vi "Create Menu Options.vi"(6 "Variant in":variant, 7 "Shift Pressed?":bool, 8 "error in (no error)":errorcluster, 10 "QD Combo Box Ref":refnum<vi>, 11 "QD Launch VI Ref":refnum<vi>) -> (0 "error out":errorcluster, 4 "Variant out":variant)   [LabVIEW 2020]
doc: "PLUGIN_DESCRIPTION: Allows you to perform all the options in the right-click > Create... menu with your keyboard. You can perform these operations with one or more objects selected.\n\nSupported options: local, reference, property, invoke, control, indicator, constant\n\nNote: there are a number of \"shorthand\" commands recognized for each object type. For example, you could type ctl instead of control. View the diagram of the plugin VI to see all supported shorthand commands (or add your own).\n\nPLUGIN_DEFAULT_SHORTCUT: a"
panel:
  in  "Undo Name":string="Object Creation"
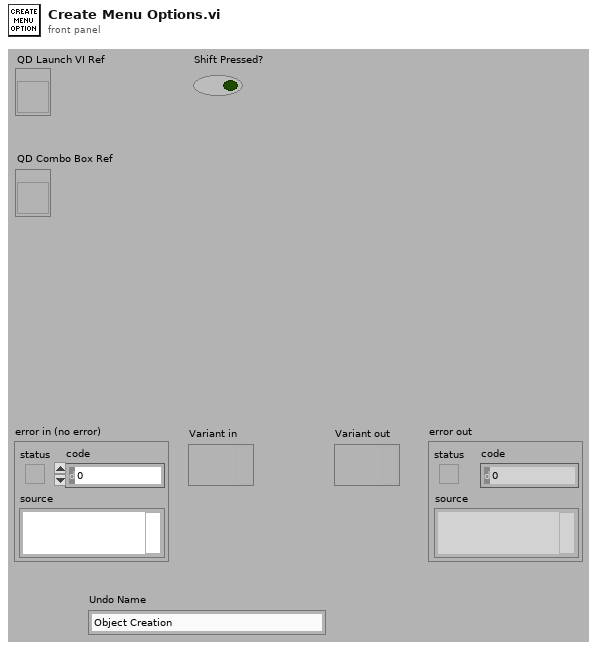
[diagram p1: front panel]
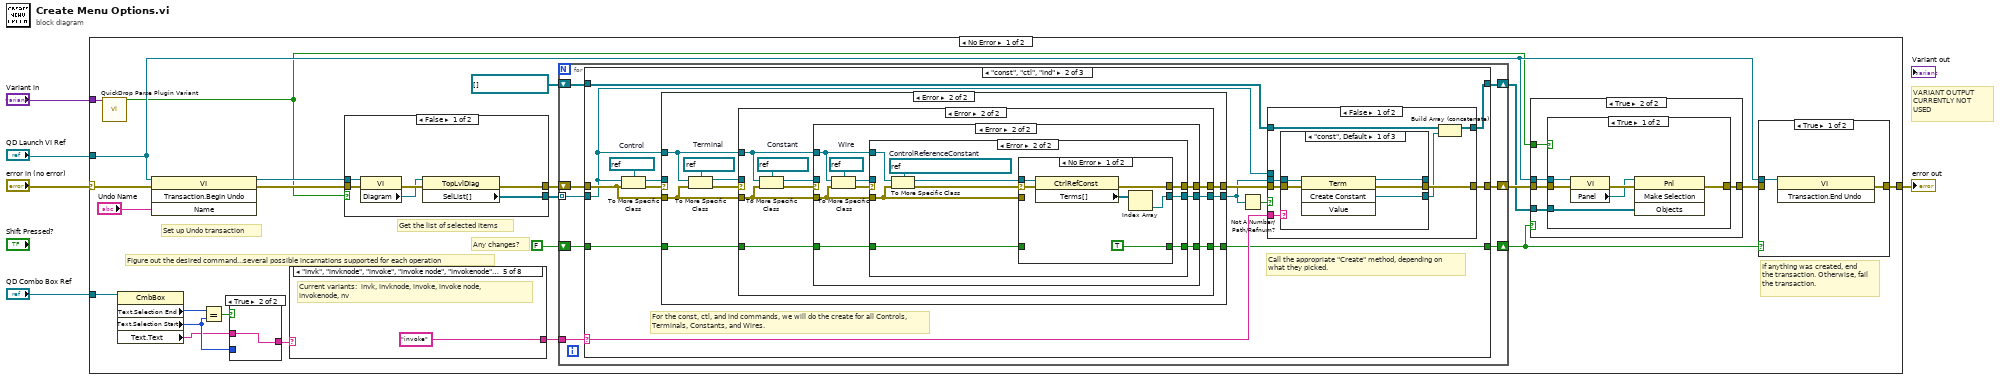
[diagram p0: block diagram]
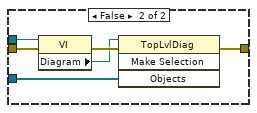
[diagram p3: hidden frame]
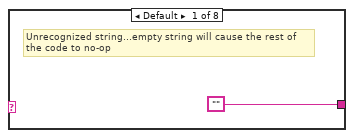
[diagram p4: hidden frame]
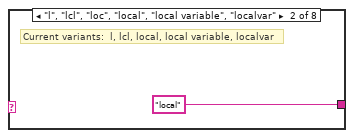
[diagram p5: hidden frame]
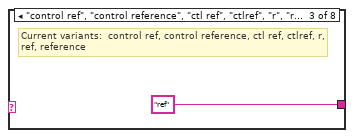
[diagram p6: hidden frame]
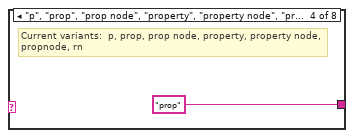
[diagram p7: hidden frame]
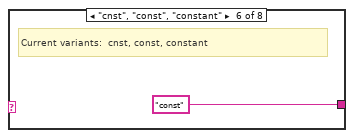
[diagram p8: hidden frame]
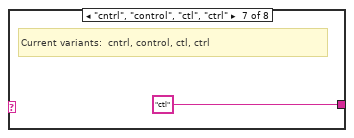
[diagram p9: hidden frame]
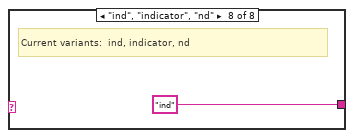
[diagram p10: hidden frame]
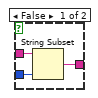
[diagram p11: hidden frame]
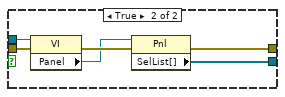
[diagram p12: hidden frame]
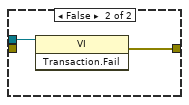
[diagram p13: hidden frame]
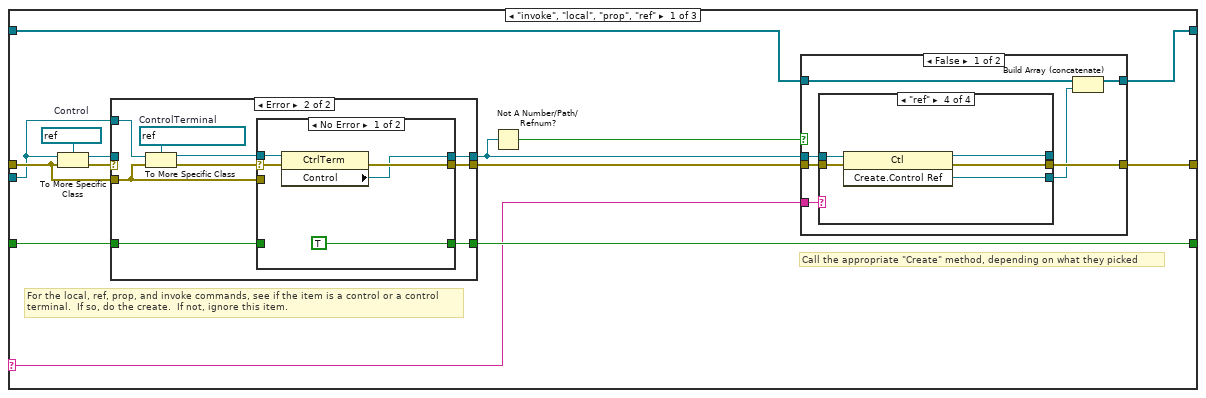
[diagram p14: hidden frame]
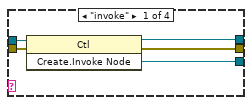
[diagram p15: hidden frame]
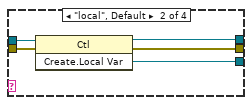
[diagram p16: hidden frame]
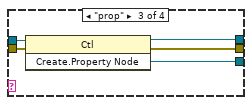
[diagram p17: hidden frame]
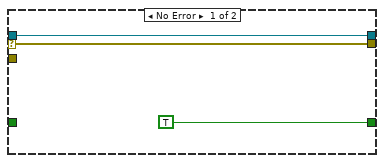
[diagram p19: hidden frame]
diagram:
  # "VARIANT OUTPUT\nCURRENTLY NOT\nUSED"
  n1 = case shown="No Error" "error in (no error)" {
    selector: "error in (no error)" -> [w27 w250]
    tunnel: [w24 w250] -> w4
    tunnel: "QD Combo Box Ref" -> [w19 _]
    tunnel: "QD Launch VI Ref" -> [w9 _]
    tunnel: "Variant in" -> [w15 _]
    frame No Error {
      # "Figure out the desired command...several possible incarnations supported for each operation"
      # "If anything was created, end the transaction. Otherwise, fail the transaction."
      # "Any changes?"
      # "Get the list of selected items"
      # "Set up Undo transaction"
      n2 = call <vilib>:"QuickDrop Parse Plugin Variant.vi"("QDKS Variant in"=w15) -> ("QD Launch VI Panel?"=w8:bool)  [unwired: 12 in, 2 out]
      n3 = property on="Property Node" class="CmbBox"(reference=w19) -> ("Text.Selection End"=w23:u32, "Text.Selection Start"=w21:u32, "Text.Text"=w20:string)  [unwired: 1 in, 2 out]
      n4 = invoke class="VI" method="Transaction.Begin Undo"(reference=w9, error in=w27, "Name"="Undo Name") -> (reference out=w13:refnum<vi>, error out=w14:errorcluster)  [unwired: 1 in, 2 out]
      n5 = Equal?(x=w23, y=w21) -> (x = y?=w22:bool)
      n6 = case shown="True" w22 {
        tunnel: [w57 w58] -> w18
        tunnel: w21 -> [w56 _]
        tunnel: w20 -> [w55 w58]
        frame False {
          n7 = String Subset(string=w55, length (rest)=w56) -> (substring=w57:string)  [unwired: 1 out]
        }
        frame True {
        }
      }
      n8 = case shown="\"invk\", \"invknode\", \"invoke\", \"invoke node\", \"invokenode\", \"nv\"" w18 {
        tunnel: ["" "local" "ref" "prop" "invoke" "const" "ctl" "ind"] -> w17
        frame Default {
          # "Unrecognized string...empty string will cause the rest of\nthe code to no-op"
        }
        frame "l", "lcl", "loc", "local", "local variable", "localvar" {
          # "Current variants:  l, lcl, local, local variable, localvar"
        }
        frame "control ref", "control reference", "ctl ref", "ctlref", "r", "ref", "reference" {
          # "Current variants:  control ref, control reference, ctl ref, ctlref, r, ref, reference"
        }
        frame "p", "prop", "prop node", "property", "property node", "propnode", "rn" {
          # "Current variants:  p, prop, prop node, property, property node, propnode, rn"
        }
        frame "invk", "invknode", "invoke", "invoke node", "invokenode", "nv" {
          # "Current variants:  invk, invknode, invoke, invoke node, invokenode, nv"
        }
        frame "cnst", "const", "constant" {
          # "Current variants:  cnst, const, constant"
        }
        frame "cntrl", "control", "ctl", "ctrl" {
          # "Current variants:  cntrl, control, ctl, ctrl"
        }
        frame "ind", "indicator", "nd" {
          # "Current variants:  ind, indicator, nd"
        }
      }
      n9 = case shown="False" w8 {
        tunnel: [w62 w68] -> w16
        tunnel: [w59 w67] -> w25
        tunnel: w14 -> [w61 w66]
        tunnel: w13 -> [w60 w65]
        frame False {
          n10 = property class="VI"(reference=w60, error in=w61) -> (error out=w64:errorcluster, "Diagram"=w63:refnum<vi>)  [unwired: 1 out]
          n11 = property class="TopLvlDiag"(reference=w63, error in=w64) -> (error out=w59:errorcluster, "SelList[]"=w62:refnum<vi>[])  [unwired: 1 out]
        }
        frame True {
          n12 = property class="VI"(reference=w65, error in=w66) -> (error out=w70:errorcluster, "Panel"=w69:refnum<vi>)  [unwired: 1 out]
          n13 = property class="Pnl"(reference=w69, error in=w70) -> (error out=w67:errorcluster, "SelList[]"=w68:refnum<vi>[])  [unwired: 1 out]
        }
      }
      n14 = for {
        tunnel: w16 -> [w78] mode=indexing
        shift-right: [w77] -> w12
        shift-left: w25 -> [w82]
        shift-right: [w79] -> w11
        shift-left: FALSE -> [w80]
        tunnel: w17 -> [w81]
        shift-right: [w75] -> w6
        shift-left: refnum<vi>[] [] -> [w76]
        n15 = case shown="\"const\", \"ctl\", \"ind\"" w81 {
          selector: w81 -> [w85 w150 _]
          tunnel: w82 -> [w94 w156 w248]
          tunnel: w78 -> [w90 w148 _]
          tunnel: w80 -> [w92 w154 w249]
          tunnel: [w91 w147 w249] -> w79
          tunnel: [w87 w151 w248] -> w77
          tunnel: w76 -> [w84 w146 w247]
          tunnel: [w83 w145 w247] -> w75
          frame "invoke", "local", "prop", "ref" {
            w96 = refnum<vi> refnum  # Control
            # "Call the appropriate \"Create\" method, depending on what they picked"
            # "For the local, ref, prop, and invoke commands, see if the item is a control or a control terminal.  If so, do the create.  If not, ignore this item."
            n16 = To More Specific Class(target class=w96, reference=w90, error in=w94) -> (specific class reference=w93:refnum<vi>, error out=w95:errorcluster)
            n17 = case shown="Error" w95 {
              selector: w95 -> [w126 _]
              tunnel: w94 -> [_ w129]
              tunnel: [w128 w130] -> w86
              tunnel: w93 -> [w128 _]
              tunnel: w92 -> [_ w133]
              tunnel: [TRUE w132] -> w91
              tunnel: w90 -> [_ w137]
              tunnel: [w126 w131] -> w88
              frame No Error {
              }
              frame Error {
                w136 = refnum<vi> refnum  # ControlTerminal
                n18 = To More Specific Class(target class=w136, reference=w137, error in=w129) -> (specific class reference=w134:refnum<vi>, error out=w135:errorcluster)
                n19 = case shown="No Error" w135 {
                  selector: w135 -> [w141 _]
                  tunnel: w134 -> [w142 _]
                  tunnel: w133 -> [_ w143]
                  tunnel: [TRUE w143] -> w132
                  tunnel: [w139 w144] -> w131
                  tunnel: [w138 _] -> w130
                  tunnel: w129 -> [_ w144]
                  frame No Error {
                    n20 = property class="CtrlTerm"(reference=w142, error in=w141) -> (error out=w139:errorcluster, "Control"=w138:refnum<vi>)  [unwired: 1 out]
                  }
                  frame Error {
                  }
                }
              }
            }
            n21 = Not A Number/Path/Refnum?(number/path/refnum=w86) -> (NaN/Path/Refnum?=w89:bool)
            n22 = case shown="False" w89 {
              tunnel: w88 -> [w102 w125]
              tunnel: [w100 w125] -> w87
              tunnel: w86 -> [w101 _]
              tunnel: w85 -> [w103 _]
              tunnel: w84 -> [w97 w124]
              tunnel: [w99 w124] -> w83
              frame False {
                n23 = case shown="\"ref\"" w103 {
                  tunnel: w102 -> [w108 w113 w118 w123]
                  tunnel: w101 -> [w107 w112 w117 w122]
                  tunnel: [w106 w111 w116 w121] -> w100
                  tunnel: [w105 w110 w115 w120] -> _
                  tunnel: [w104 w109 w114 w119] -> w98
                  frame "invoke" {
                    n24 = invoke class="Ctl" method="Create.Invoke Node"(reference=w107, error in=w108) -> (reference out=w105:refnum<vi>, error out=w106:errorcluster, "Create Invoke Node"=w104:refnum<vi>)  [unwired: 1 in]
                  }
                  frame "local", Default {
                    n25 = invoke class="Ctl" method="Create.Local Var"(reference=w112, error in=w113) -> (reference out=w110:refnum<vi>, error out=w111:errorcluster, "Create Local"=w109:refnum<vi>)  [unwired: 1 in]
                  }
                  frame "prop" {
                    n26 = invoke class="Ctl" method="Create.Property Node"(reference=w117, error in=w118) -> (reference out=w115:refnum<vi>, error out=w116:errorcluster, "Create Property Node"=w114:refnum<vi>)  [unwired: 1 in]
                  }
                  frame "ref" {
                    n27 = invoke class="Ctl" method="Create.Control Ref"(reference=w122, error in=w123) -> (reference out=w120:refnum<vi>, error out=w121:errorcluster, "Create Control Ref"=w119:refnum<vi>)  [unwired: 1 in]
                  }
                }
                n28 = Build Array (concatenate)(w97, w98) -> (w99:refnum<vi>[])
              }
              frame True {
              }
            }
          }
          frame "const", "ctl", "ind" {
            w158 = refnum<vi> refnum  # Control
            # "Call the appropriate \"Create\" method, depending on what they picked."
            # "For the const, ctl, and ind commands, we will do the create for all Controls, Terminals, Constants, and Wires."
            n29 = To More Specific Class(target class=w158, reference=w148, error in=w156) -> (specific class reference=w155:refnum<vi>, error out=w157:errorcluster)
            n30 = case shown="Error" w157 {
              selector: w157 -> [w186 _]
              tunnel: w156 -> [_ w190]
              tunnel: w155 -> [w185 _]
              tunnel: w154 -> [_ w193]
              tunnel: [TRUE w192] -> w147
              tunnel: w148 -> [_ w188]
              tunnel: [w184 w191] -> w152
              tunnel: [w183 w189] -> w149
              frame No Error {
                n31 = property class="Ctl"(reference=w185, error in=w186) -> (error out=w184:errorcluster, "Terminal"=w183:refnum<vi>)  [unwired: 1 out]
              }
              frame Error {
                w196 = refnum<vi> refnum  # Terminal
                n32 = To More Specific Class(target class=w196, reference=w188, error in=w190) -> (specific class reference=w194:refnum<vi>, error out=w195:errorcluster)
                n33 = case shown="Error" w195 {
                  selector: w195 -> [w198 _]
                  tunnel: w194 -> [w197 _]
                  tunnel: w193 -> [_ w202]
                  tunnel: [TRUE w201] -> w192
                  tunnel: [w198 w203] -> w191
                  tunnel: w190 -> [_ w206]
                  tunnel: [w197 w204] -> w189
                  tunnel: w188 -> [_ w200]
                  frame No Error {
                  }
                  frame Error {
                    w208 = refnum<vi> refnum  # Constant
                    n34 = To More Specific Class(target class=w208, reference=w200, error in=w206) -> (specific class reference=w205:refnum<vi>, error out=w207:errorcluster)
                    n35 = case shown="Error" w207 {
                      selector: w207 -> [w213 _]
                      tunnel: w206 -> [_ w217]
                      tunnel: w205 -> [w212 _]
                      tunnel: [w211 w218] -> w204
                      tunnel: [w210 w219] -> w203
                      tunnel: w202 -> [_ w216]
                      tunnel: [TRUE w215] -> w201
                      tunnel: w200 -> [_ w214]
                      frame No Error {
                        n36 = property class="Const"(reference=w212, error in=w213) -> (error out=w210:errorcluster, "Terminal"=w211:refnum<vi>)  [unwired: 1 out]
                      }
                      frame Error {
                        w222 = refnum<vi> refnum  # Wire
                        n37 = To More Specific Class(target class=w222, reference=w214, error in=w217) -> (specific class reference=w220:refnum<vi>, error out=w221:errorcluster)
                        n38 = case shown="Error" w221 {
                          selector: w221 -> [w229 _]
                          tunnel: w220 -> [w228 _]
                          tunnel: [w227 w232] -> w219
                          tunnel: [w224 w230] -> w218
                          tunnel: w217 -> [_ w231]
                          tunnel: w216 -> [_ w234]
                          tunnel: [TRUE w233] -> w215
                          tunnel: w214 -> [_ w237]
                          frame No Error {
                            n39 = property class="Wire"(reference=w228, error in=w229) -> (error out=w227:errorcluster, "Terms[]"=w226:refnum<vi>[])  [unwired: 1 out]
                            n40 = Delete From Array(array=w226, index=0) -> (deleted portion=w224:refnum<vi>)  [unwired: 1 in, 1 out]
                          }
                          frame Error {
                            w238 = refnum<vi> refnum  # ControlReferenceConstant
                            n41 = To More Specific Class(target class=w238, reference=w237, error in=w231) -> (specific class reference=w236:refnum<vi>, error out=w235:errorcluster)
                            n42 = case shown="No Error" w235 {
                              selector: w235 -> [w243 _]
                              tunnel: w236 -> [w242 _]
                              tunnel: w234 -> [_ w246]
                              tunnel: [TRUE w246] -> w233
                              tunnel: [w241 w245] -> w232
                              tunnel: w231 -> [_ w245]
                              tunnel: [w239 _] -> w230
                              frame No Error {
                                n43 = property class="CtrlRefConst"(reference=w242, error in=w243) -> (error out=w241:errorcluster, "Terms[]"=w240:refnum<vi>[])  [unwired: 1 out]
                                n44 = Index Array(array=w240) -> (element=w239:refnum<vi>)  [unwired: 1 in]
                              }
                              frame Error {
                              }
                            }
                          }
                        }
                      }
                    }
                  }
                }
              }
            }
            n45 = Not A Number/Path/Refnum?(number/path/refnum=w149) -> (NaN/Path/Refnum?=w153:bool)
            n46 = case shown="False" w153 {
              tunnel: w152 -> [w164 w182]
              tunnel: [w162 w182] -> w151
              tunnel: w149 -> [w163 _]
              tunnel: w150 -> [w165 _]
              tunnel: w148 -> [_ _]
              tunnel: w146 -> [w161 w181]
              tunnel: [w160 w181] -> w145
              frame False {
                n47 = case shown="\"const\", Default" w165 {
                  tunnel: w164 -> [w170 w175 w180]
                  tunnel: w163 -> [w169 w174 w179]
                  tunnel: [w168 w173 w178] -> w162
                  tunnel: [w167 w172 w177] -> _
                  tunnel: [w166 w171 w176] -> w159
                  frame "const", Default {
                    n48 = invoke class="Term" method="Create Constant"(reference=w169, error in=w170) -> (reference out=w167:refnum<vi>, error out=w168:errorcluster, "Create Constant"=w166:refnum<vi>)  [unwired: 2 in, 1 out]
                  }
                  frame "ctl" {
                    n49 = invoke class="Term" method="Create Control"(reference=w174, error in=w175) -> (reference out=w172:refnum<vi>, error out=w173:errorcluster, "Create Control"=w171:refnum<vi>)  [unwired: 2 in, 1 out]
                  }
                  frame "ind" {
                    n50 = invoke class="Term" method="Create Indicator"(reference=w179, error in=w180) -> (reference out=w177:refnum<vi>, error out=w178:errorcluster, "Create Indicator"=w176:refnum<vi>)  [unwired: 1 in]
                  }
                }
                n51 = Build Array (concatenate)(w161, w159) -> (w160:refnum<vi>[])
              }
              frame True {
              }
            }
          }
          frame "", Default {
            # "Unrecognized command...do nothing"
          }
        }
      }
      n52 = case shown="True" w11 {
        tunnel: w12 -> [w29 w34]
        tunnel: [w29 w31] -> w10
        tunnel: w9 -> [_ w32]
        tunnel: w8 -> [_ w33]
        tunnel: w6 -> [_ w30]
        frame False {
        }
        frame True {
          n53 = case shown="True" w33 {
            tunnel: w34 -> [w40 w46]
            tunnel: w32 -> [w39 w45]
            tunnel: [w36 w42] -> w31
            tunnel: w30 -> [w35 w41]
            frame True {
              n54 = property class="VI"(reference=w39, error in=w40) -> (error out=w38:errorcluster, "Panel"=w37:refnum<vi>)  [unwired: 1 out]
              n55 = invoke class="Pnl" method="Make Selection"(reference=w37, error in=w38, "Objects"=w35) -> (error out=w36:errorcluster)  [unwired: 1 in, 3 out]
            }
            frame False {
              n56 = property class="VI"(reference=w45, error in=w46) -> (error out=w44:errorcluster, "Diagram"=w43:refnum<vi>)  [unwired: 1 out]
              n57 = invoke class="TopLvlDiag" method="Make Selection"(reference=w43, error in=w44, "Objects"=w41) -> (error out=w42:errorcluster)  [unwired: 1 in, 3 out]
            }
          }
        }
      }
      n58 = case shown="True" w11 {
        tunnel: w9 -> [w71 w73]
        tunnel: [w72 w74] -> w24
        tunnel: w10 -> [_ _]
        frame True {
          n59 = invoke class="VI" method="Transaction.End Undo"(reference=w71) -> (error out=w72:errorcluster)  [unwired: 2 in, 2 out]
        }
        frame False {
          n60 = invoke class="VI" method="Transaction.Fail"(reference=w73) -> (error out=w74:errorcluster)  [unwired: 2 in, 2 out]
        }
      }
    }
    frame Error {
    }
  }
  "error out" <- w4
